vi "Agilent 34401 Acquire and Chart - Triggered.vi"() -> ()   [LabVIEW 2022 SP3]
doc: "This example shows how to configure an immediately or externally triggered measurement using the low-level Data VIs to retrieve data from the DMM. Measurements are sent directly to the instrument's output buffer where they are read iteratively and charted.\n\n<B>Note:</B>\n\n(1) This example does <B>not</B> support software triggering.\n\n(2) External triggers are not processed while the instrument is acquiring samples.\n\n(3) It is recommended that all triggered measurements be made using an appropriate fixed manual range. That is, disable autorange and manually select a range in <B>Configure Measurement VI</B>.\n\n(4) To increase the speed of DC measurements, set Autozero to \"once,\" or \"off\" in <B>Configure Autozero VI</B>. \n\n(5) For faster AC measurements, call <B>Configure AC Filter VI</B> to set the AC filter to 200 Hz, and set the manual trigger delay to 0 seconds in <B>Configure Trigger VI</B>."
uses:
  <vilib>/Utility/error.llb/DialogType.ctl
  <instrlib>/Agilent 34401/Agilent 34401.lvlib
panel:
  in  "Function (0: DC Voltage)":u16(ring) items=["DC Voltage", "AC Voltage", "2 - Wire Resistance", "4 - Wire Resistance", "DC Current", "AC Current", "Frequency", "Period", "Continuity", "Diode Checking", "VDC:VDC Ratio", "Temperature", "Capacitance"]
  in  "Trigger Source (0: Immediate)":u16(ring) items=["Immediate", "Software (Bus)", "External", "Internal"]
  in  "Manual Range (1.00)":dbl=1.0 format="%_3f"
  in  "Enable Auto Range (F: Disable)":bool
  in  "Trigger Count (5)":i32=5 format="%#.6g"
  in  "Stop":bool
  out "Trigger Iteration":i32
  in  "Samples per Trigger (10)":i32=10 format="%#.6g"
  in  "Timeout (10000 ms)":u32=10000
  out "Measurements":dbl[](graph)=[0.002500734, 0.002496723, 0.002491019, 0.002484271, 0.002477294]
  in  "VISA resource name":refnum<visa-resource-name>
  # "(c) 2005-2015 National Instruments.  ALL RIGHTS RESERVED."
  # "Note: Software triggering is not\nsupported  in this example."
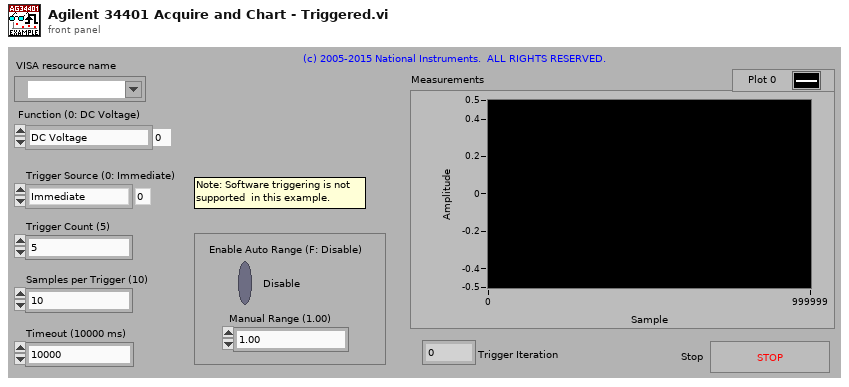
[diagram p1: front panel]
types:
  T1 = typedef "DialogType.ctl" = u16
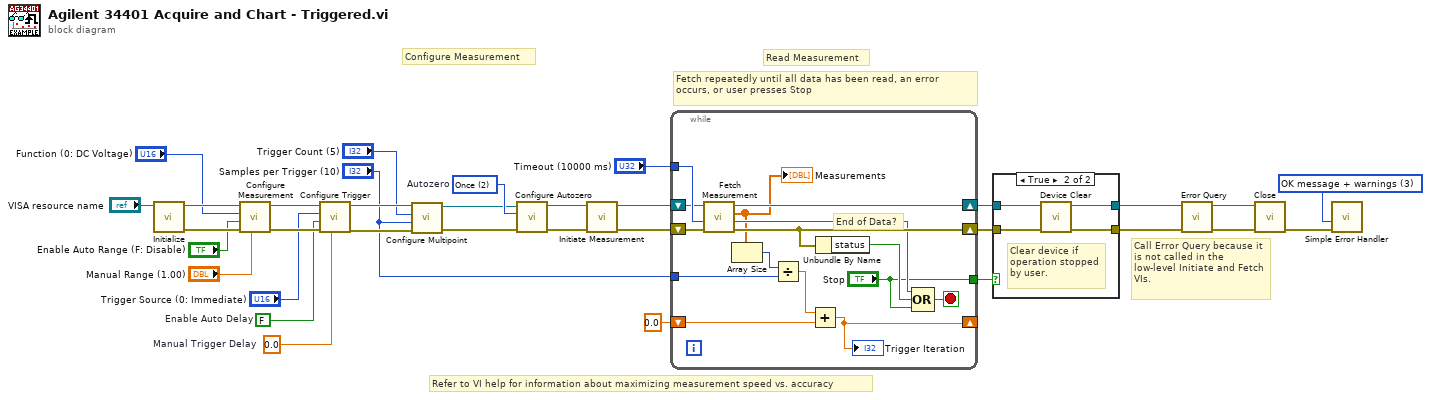
[diagram p0: block diagram]
diagram:
  w2 = 0.0  # Manual Trigger Delay
  w3 = FALSE  # Enable Auto Delay
  w11 = T1 3 items=["no dialog", "OK message", "continue or stop message", "OK message + warnings", "continue/stop + warnings"] ("type of dialog (OK msg:1)")
  w29 = u16 2 items=["On", "Off", "Once"]  # Autozero
  # "Call Error Query because it is not called in the low-level Initiate and Fetch VIs."
  # "Fetch repeatedly until all data has been read, an error occurs, or user presses Stop"
  # "Refer to VI help for information about maximizing measurement speed vs. accuracy"
  # "Read Measurement"
  # "Configure Measurement"
  n1 = call <instrlib>:"Initialize.vi"("VISA resource name"="VISA resource name") -> ("error out"=w30:errorcluster, "VISA resource name out"=w31:refnum<visa-resource-name>)  [unwired: 9 in]
  n2 = call <instrlib>:"Configure Measurement.vi"("Manual Range (1.00)"="Manual Range (1.00)", "error in (no error)"=w30, "Enable Auto Range (T: Enable)"="Enable Auto Range (F: Disable)", "Function (0: DC Voltage)"="Function (0: DC Voltage)", "VISA resource name"=w31) -> ("error out"=w22:errorcluster, "VISA resource name out"=w23:refnum<visa-resource-name>)  [unwired: 5 in]
  n3 = call <instrlib>:"Configure Trigger.vi"("Manual Trigger Delay (0.0 s)"=w2, "error in (no error)"=w22, "Enable Auto Delay (T: Enable)"=w3, "Trigger Source (0: Immediate)"="Trigger Source (0: Immediate)", "VISA resource name"=w23) -> ("error out"=w20:errorcluster, "VISA resource name out"=w21:refnum<visa-resource-name>)  [unwired: 5 in]
  n4 = call <instrlib>:"Configure Multipoint.vi"("error in (no error)"=w20, "Sample Count (1)"="Samples per Trigger (10)", "Trigger Count (1)"="Trigger Count (5)", "VISA resource name"=w21) -> ("error out"=w26:errorcluster, "VISA resource name out"=w27:refnum<visa-resource-name>)  [unwired: 6 in]
  n5 = call <instrlib>:"Configure Autozero.vi"("error in (no error)"=w26, "Autozero  (0: On)"=w29, "VISA resource name"=w27) -> ("error out"=w18:errorcluster, "VISA resource name out"=w19:refnum<visa-resource-name>)  [unwired: 7 in]
  n6 = call <instrlib>:"Initiate Measurement.vi"("error in (no error)"=w18, "VISA resource name"=w19) -> ("error out"=w16:errorcluster, "VISA resource name out"=w17:refnum<visa-resource-name>)  [unwired: 8 in]
  n7 = while {
    tunnel: "Timeout (10000 ms)" -> [w47]
    shift-right: [w43] -> w24
    shift-left: w16 -> [w45]
    shift-right: [w48] -> w25
    shift-left: w17 -> [w46]
    tunnel: ["Stop"] -> w15
    tunnel: "Samples per Trigger (10)" -> [w37]
    shift-right: [w35] -> _
    shift-left: 0.0 -> [w34]
    stop <- w44 stop-if-true
    # "End of Data?"
    n8 = call <instrlib>:"Fetch Measurement.vi"("error in (no error)"=w45, "Timeout (10000 ms)"=w47, "VISA resource name"=w46) -> ("error out"=w43:errorcluster, "End of Data?"=w41:bool, "Measurements"=w39:dbl[], "VISA resource name out"=w48:refnum<visa-resource-name>)  [unwired: 5 in]
    "Measurements" <- w39
    n9 = Array Size(array=w39) -> (size(s)=w38:i32)
    n10 = Divide(x=w38, y=w37) -> (x/y=w36:dbl)
    n11 = Add(x=w36, y=w34) -> (x+y=w35:dbl)
    "Trigger Iteration" <- w35
    n12 = Unbundle By Name(w43) -> ("status"=w42:bool)
    n13 = Compound Arithmetic op=OR(w41, w42, "Stop") -> (w44:bool)
  }
  n14 = case shown="True" w15 {
    tunnel: w25 -> [w50 w54]
    tunnel: w24 -> [w49 w53]
    tunnel: [w50 w52] -> w6
    tunnel: [w49 w51] -> w5
    frame False {
    }
    frame True {
      # "Clear device if operation stopped by user."
      n15 = call <instrlib>:"Device Clear.vi"("error in (no error)"=w53, "VISA Resource Name"=w54) -> ("error out"=w51:errorcluster, "VISA Resource Out"=w52:refnum<visa-resource-name>)  [unwired: 8 in]
    }
  }
  n16 = call <instrlib>:"Error Query.vi"("error in (no error)"=w5, "VISA resource name"=w6) -> ("error out"=w8:errorcluster, "VISA resource name out"=w7:refnum<visa-resource-name>)  [unwired: 6 in, 2 out]
  n17 = call <instrlib>:"Close.vi"("error in (no error)"=w8, "VISA resource name"=w7) -> ("error out"=w33:errorcluster)  [unwired: 9 in]
  n18 = call <vilib>:"Simple Error Handler.vi"("type of dialog (OK msg:1)"=w11, "error in (no error)"=w33) -> ()  [unwired: 3 in, 5 out]
